vi "DecodeReadMessage.vi"(5 "Message":string) -> (0 "Value":i32, 1 "Key":u32, 2 "Device":u8)   [LabVIEW 2021]
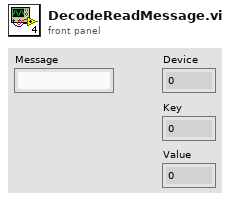
[diagram p1: front panel]
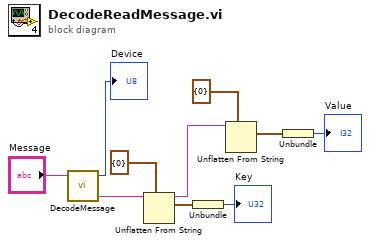
[diagram p0: block diagram]
diagram:
  n1 = call "DecodeMessage.vi"("Message"="Message") -> ("Payload"=w8:string, "Device"=→"Device":u8)  [unwired: 2 in, 1 out]
  n2 = Unflatten From String(type=cluster{u32} {0}, binary string=w8) -> (rest of the binary string=w7:string, value=w5:cluster{u32})  [unwired: 3 in, 1 out]
  n3 = Unbundle(w5) -> (→"Key":u32)
  n4 = Unflatten From String(type=cluster{i32} {0}, binary string=w7) -> (value=w3:cluster{i32})  [unwired: 3 in, 2 out]
  n5 = Unbundle(w3) -> (→"Value":i32)
